vi "Add FPGA Sections.vi"(8 "error in (no error)":errorcluster, 11 "Node Ptr":T1 format="%.0x") -> (0 "error out":errorcluster, 3 "Parent Ref out":T1 format="%.0x")   [LabVIEW 2016, in "FPGA Addon System Explorer.lvlib"]
uses:
  FPGA Addon System Explorer.lvlib
  <vilib>/NI Veristand/Custom Device API/Custom Device Item Ref.ctl
  Shared/Constants.vi
  <vilib>/NI VeriStand/Custom Device API/Custom Device API.lvlib
  Shared/FPGA Addon Shared.lvlib
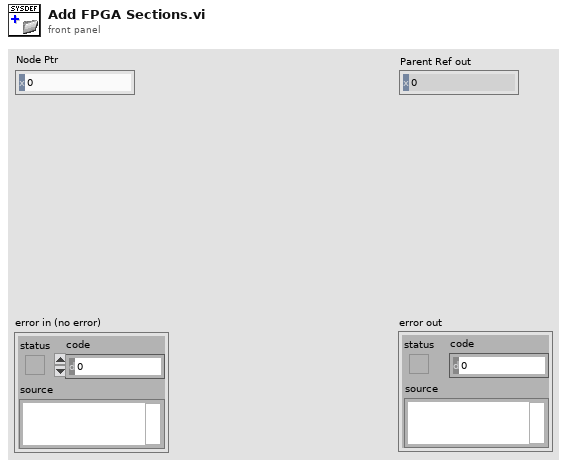
[diagram p1: front panel]
types:
  T1 = typedef "Custom Device API.lvlib/Custom Device Item Ref.ctl" = u64
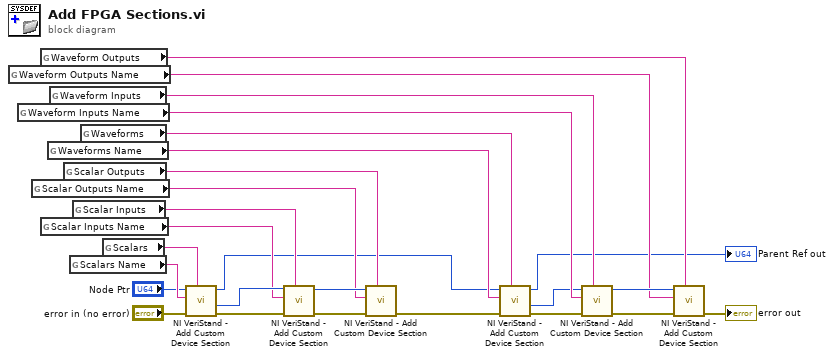
[diagram p0: block diagram]
diagram:
  n1 = global read "Constants.vi" "Waveform Outputs Name"() -> (w6:string)
  n2 = global read "Constants.vi" "Waveform Inputs Name"() -> (w13:string)
  n3 = global read "Constants.vi" "Scalar Outputs Name"() -> (w18:string)
  n4 = global read "Constants.vi" "Waveform Outputs"() -> (w5:string)
  n5 = global read "Constants.vi" "Scalar Inputs Name"() -> (w22:string)
  n6 = global read "Constants.vi" "Waveforms Name"() -> (w16:string)
  n7 = global read "Constants.vi" "Waveform Inputs"() -> (w12:string)
  n8 = global read "Constants.vi" "Scalar Outputs"() -> (w17:string)
  n9 = global read "Constants.vi" "Scalars Name"() -> (w25:string)
  n10 = global read "Constants.vi" "Scalar Inputs"() -> (w21:string)
  n11 = global read "Constants.vi" "Waveforms"() -> (w15:string)
  n12 = global read "Constants.vi" "Scalars"() -> (w26:string)
  n13 = call <vilib>:"NI VeriStand - Add Custom Device Section.vi"("GUID (Default Section)"=w26, "error in (no error)"="error in (no error)", "Section Name"=w25, "Parent Ref in"="Node Ptr") -> ("error out"=w24:errorcluster, "Section Ptr"=w23:T1, "Parent Ref out"=w11:T1)  [unwired: 4 in, 1 out]
  n14 = call <vilib>:"NI VeriStand - Add Custom Device Section.vi"("GUID (Default Section)"=w21, "error in (no error)"=w24, "Section Name"=w22, "Parent Ref in"=w23) -> ("error out"=w19:errorcluster, "Parent Ref out"=w20:T1)  [unwired: 4 in, 2 out]
  n15 = call <vilib>:"NI VeriStand - Add Custom Device Section.vi"("GUID (Default Section)"=w17, "error in (no error)"=w19, "Section Name"=w18, "Parent Ref in"=w20) -> ("error out"=w10:errorcluster)  [unwired: 4 in, 3 out]
  n16 = call <vilib>:"NI VeriStand - Add Custom Device Section.vi"("GUID (Default Section)"=w15, "error in (no error)"=w10, "Section Name"=w16, "Parent Ref in"=w11) -> ("error out"=w14:errorcluster, "Section Ptr"=w7:T1, "Parent Ref out"=→"Parent Ref out":T1)  [unwired: 4 in, 1 out]
  n17 = call <vilib>:"NI VeriStand - Add Custom Device Section.vi"("GUID (Default Section)"=w12, "error in (no error)"=w14, "Section Name"=w13, "Parent Ref in"=w7) -> ("error out"=w8:errorcluster, "Parent Ref out"=w9:T1)  [unwired: 4 in, 2 out]
  n18 = call <vilib>:"NI VeriStand - Add Custom Device Section.vi"("GUID (Default Section)"=w5, "error in (no error)"=w8, "Section Name"=w6, "Parent Ref in"=w9) -> ("error out"=→"error out":errorcluster)  [unwired: 4 in, 3 out]
